vi "getAll.vi"(8 "error in (no error)":errorcluster, 11 "Instrument.VRM in":refnum<class "Instrument.OxfordVRM.lvclass">) -> (0 "error out":errorcluster, 2 "getAll":variant, 3 "Instrument.VRM out":refnum<class "Instrument.OxfordVRM.lvclass">)   [LabVIEW 2019, in "Instrument.OxfordVRM.lvclass"]
uses:
  Instrument.OxfordVRM.lvclass
  <userlib>/LevyLab/Levylab Instruments/Instrument Types/Cryostat/Typedefs/Magnet Axis--Enum.ctl
  Instrument.OxfordVRM.lvclass/Instrument.OxfordVRM.ctl
  <userlib>/LevyLab/Levylab Instruments/Instrument Types/Cryostat/Instrument.Cryostat.lvclass
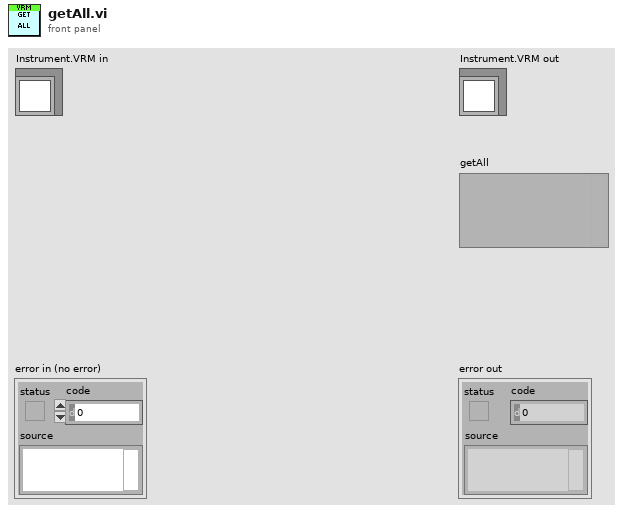
[diagram p1: front panel]
types:
  T1 = typedef "Instrument.Cryostat.lvclass/Magnet Axis--Enum.ctl" = enum16{"Z", "X", "Y"}
  T2 = typedef "Instrument.OxfordVRM.lvclass/getAll.ctl" = cluster{"Field":dbl[], "Target Field":dbl[], "Target Field Rate":dbl[], "PSU Current":dbl[], "PSU Voltage":dbl[], "Status":string[]}
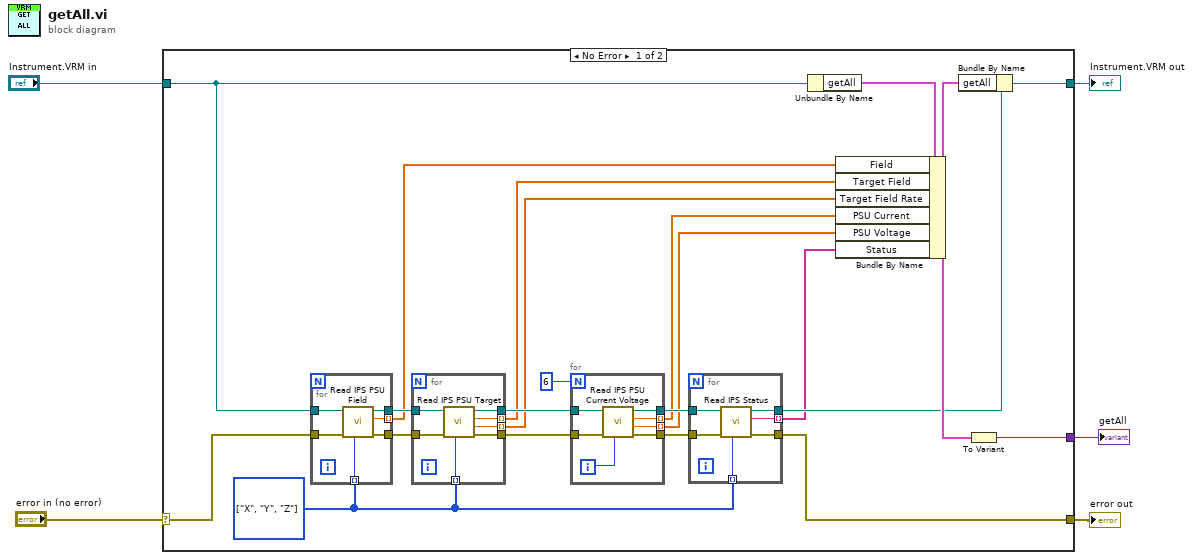
[diagram p0: block diagram]
diagram:
  n1 = case shown="No Error" "error in (no error)" {
    selector: "error in (no error)" -> [w19 w54]
    tunnel: "Instrument.VRM in" -> [w18 w55]
    tunnel: [w26 w55] -> w4
    tunnel: [w8 w54] -> w2
    tunnel: [w25 _] -> w1
    frame No Error {
      w7 = T1[] [enum."X", enum."Y", enum."Z"] items=["Z", "X", "Y"]
      n2 = for {
        tunnel: w18 -> [w39]
        tunnel: w19 -> [w38]
        tunnel: [w37] -> w14 mode=indexing
        tunnel: [w36] -> w21
        tunnel: [w35] -> w22
        tunnel: w7 -> [w34] mode=indexing
        n3 = call "Read IPS PSU Field.vi"("Axis"=w34, "error in (no error)"=w38, "Instrument.OxfordVRM in"=w39) -> ("error out"=w36:errorcluster, "Power Supply Field (T)"=w37:dbl, "Instrument.OxfordVRM out"=w35:refnum<class "Instrument.OxfordVRM.lvclass">)  [unwired: 6 in]
      }
      n4 = for {
        tunnel: w22 -> [w46]
        tunnel: w21 -> [w45]
        tunnel: [w44] -> w13 mode=indexing
        tunnel: [w43] -> w12 mode=indexing
        tunnel: [w42] -> w23
        tunnel: [w41] -> w20
        tunnel: w7 -> [w40] mode=indexing
        n5 = call "Read IPS PSU Target.vi"("Axis"=w40, "error in (no error)"=w45, "Instrument.OxfordVRM in"=w46) -> ("error out"=w41:errorcluster, "Target Field Rate (T/min)"=w43:dbl, "Target Field (T)"=w44:dbl, "Instrument.OxfordVRM out"=w42:refnum<class "Instrument.OxfordVRM.lvclass">)  [unwired: 5 in]
      }
      n6 = for {
        N: 6 -> [_]
        tunnel: w23 -> [w53]
        tunnel: w20 -> [w52]
        tunnel: [w50] -> w11 mode=indexing
        tunnel: [w49] -> w10 mode=indexing
        tunnel: [w48] -> w17
        tunnel: [w47] -> w16
        i -> [w51]
        n7 = call "Read IPS PSU Current Voltage.vi"("PSU #"=w51, "error in (no error)"=w52, "Instrument.OxfordVRM in"=w53) -> ("error out"=w47:errorcluster, "Voltage (V)"=w49:dbl, "Current (A)"=w50:dbl, "Instrument.OxfordVRM out"=w48:refnum<class "Instrument.OxfordVRM.lvclass">)  [unwired: 5 in]
      }
      n8 = for {
        tunnel: w17 -> [w33]
        tunnel: w16 -> [w32]
        tunnel: [w31] -> w9 mode=indexing
        tunnel: [w30] -> w15
        tunnel: [w29] -> w8
        tunnel: w7 -> [w28] mode=indexing
        n9 = call "Read IPS Status.vi"("Axis"=w28, "error in (no error)"=w32, "Instrument.OxfordVRM in"=w33) -> ("error out"=w29:errorcluster, "Status"=w31:string, "Instrument.OxfordVRM out"=w30:refnum<class "Instrument.OxfordVRM.lvclass">)  [unwired: 6 in]
      }
      n10 = Unbundle By Name(w18) -> ("getAll"=w27:T2)
      n11 = Bundle By Name(cluster=w27, "Field"=w14, "Target Field"=w13, "Target Field Rate"=w12, "PSU Current"=w11, "PSU Voltage"=w10, "Status"=w9) -> (w24:T2)
      n12 = Bundle By Name(cluster=w15, "getAll"=w24) -> (w26:refnum<class "Instrument.OxfordVRM.lvclass">)
      n13 = To Variant(anything=w24) -> (Variant=w25:variant)
    }
    frame Error {
    }
  }
  "error out" <- w2
  "Instrument.VRM out" <- w4
  "getAll" <- w1
